vi "Close All Connections.vi"(7 "Name":string, 8 "error in":errorcluster, 11 "TCP Refs":T1) -> (0 "error out":errorcluster)   [LabVIEW 2015, in "Instrument Addon Engine.lvlib"]
uses:
  Instrument Addon Engine.lvlib
  Types/TCP Refs.ctl
  <vilib>/NI/STM/Connection Manager/TCP/Advanced/TCP Connection Manager Reference.ctl
  <vilib>/NI/STM/Connection Manager/TCP/Advanced/TCP Connection Manager State Variables.ctl
  <vilib>/NI/STM/TCP/TCP Connection Info.ctl
  <vilib>/NI/STM/SubVIs/MetaDataElement.ctl
  <vilib>/NI/STM/Connection Manager/TCP/TCP Connection Properties.ctl
  <vilib>/NI/STM/Connection Manager/TCP/TCP Connection Method.ctl
  <vilib>/NI Veristand/Custom Device Tools/Custom Device Utility Library/Custom Device Utility Library.lvlib
  <vilib>/NI/STM/NI STM.lvlib
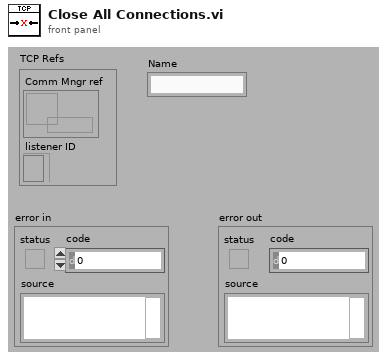
[diagram p1: front panel]
types:
  T1 = typedef "Instrument Addon Engine.lvlib/TCP Refs.ctl" = cluster{"Comm Mngr ref":T2, "listener ID":refnum<k5>}
  T2 = typedef "TCP Connection Manager Reference.ctl" = refnum<data-value>
  T3 = typedef "NI STM.lvlib/TCP Connection Method.ctl" = enum16{"Initialize", "Add Connection", "Set Properties", "Get Connection(s)", "Remove Connection", "Remove All Connections", "Get Connection Count"}
  T4 = typedef "NI STM.lvlib/TCP Connection Info.ctl" = cluster{"connection ID":refnum<k5>, "meta data":T5[]}
  T5 = typedef "NI STM.lvlib/MetaDataElement.ctl" = string
  T6 = typedef "NI STM.lvlib/TCP Connection Properties.ctl" = cluster{"Name":string, "Address":string, "Custom":string}
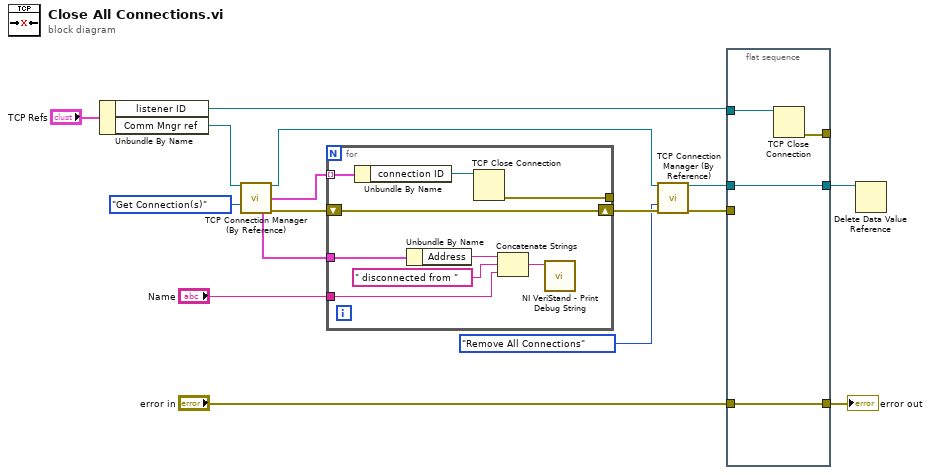
[diagram p0: block diagram]
diagram:
  n1 = Unbundle By Name("TCP Refs") -> ("listener ID"=w3:refnum<k5>, "Comm Mngr ref"=w4:T2)
  n2 = call <vilib>:"TCP Connection Manager (By Reference).vi"("connection manager ref in"=w4, "method"=TCP_Connection_Method."Get Connection(s)") -> ("connection manager ref out"=w8:T2, "all connections"=w14:T4[], "properties out"=w6:T6, "error out"=w13:errorcluster)  [unwired: 7 in, 3 out]
  n3 = for {
    tunnel: w14 -> [w17] mode=indexing
    shift-right: [w23] -> w12
    shift-left: w13 -> [w23]
    tunnel: [w24] -> _
    tunnel: "Name" -> [w19]
    tunnel: w6 -> [w18]
    n4 = Unbundle By Name(w17) -> ("connection ID"=w25:refnum<k5>)
    n5 = Unbundle By Name(w18) -> ("Address"=w20:string)
    n6 = TCP Close Connection(connection ID=w25) -> (error out=w24:errorcluster)  [unwired: 2 in, 1 out]
    n7 = Concatenate Strings(w20, " disconnected from " ("string"), w19) -> (w22:string)
    n8 = call <vilib>:"NI VeriStand - Print Debug String.vi"("Message"=w22) -> ()  [unwired: 10 in, 1 out]
  }
  n9 = call <vilib>:"TCP Connection Manager (By Reference).vi"("connection manager ref in"=w8, "method"=TCP_Connection_Method."Remove All Connections", "error in"=w12) -> ("connection manager ref out"=w10:T2, "error out"=w11:errorcluster)  [unwired: 6 in, 5 out]
  n10 = flat-sequence {
    tunnel: w3 -> [w29]
    tunnel: [w28] -> w16
    tunnel: w11 -> [_]
    tunnel: "error in" -> [w28]
    tunnel: [w27] -> _
    tunnel: w10 -> [w26]
    tunnel: [w26] -> w9
    frame #0 {
      n11 = TCP Close Connection(connection ID=w29) -> (error out=w27:errorcluster)  [unwired: 2 in, 1 out]
    }
  }
  n12 = Delete Data Value Reference(data value reference=w9) -> ()  [unwired: 1 in, 2 out]
  "error out" <- w16
